vi "删除第一个元素.vi"(2 "数组－数值 2":dbl[](array[numeric]), 3 "数组－数值":dbl[](array[numeric])) -> (0 "数组－数值 3":dbl[](array[numeric]), 1 "数组":dbl[](array[numeric]))   [LabVIEW 2016]
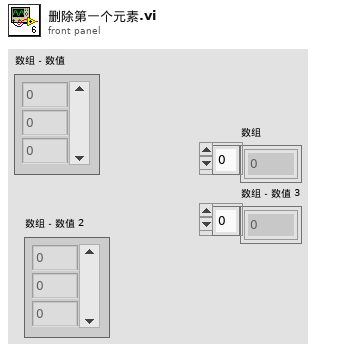
[diagram p1: front panel]
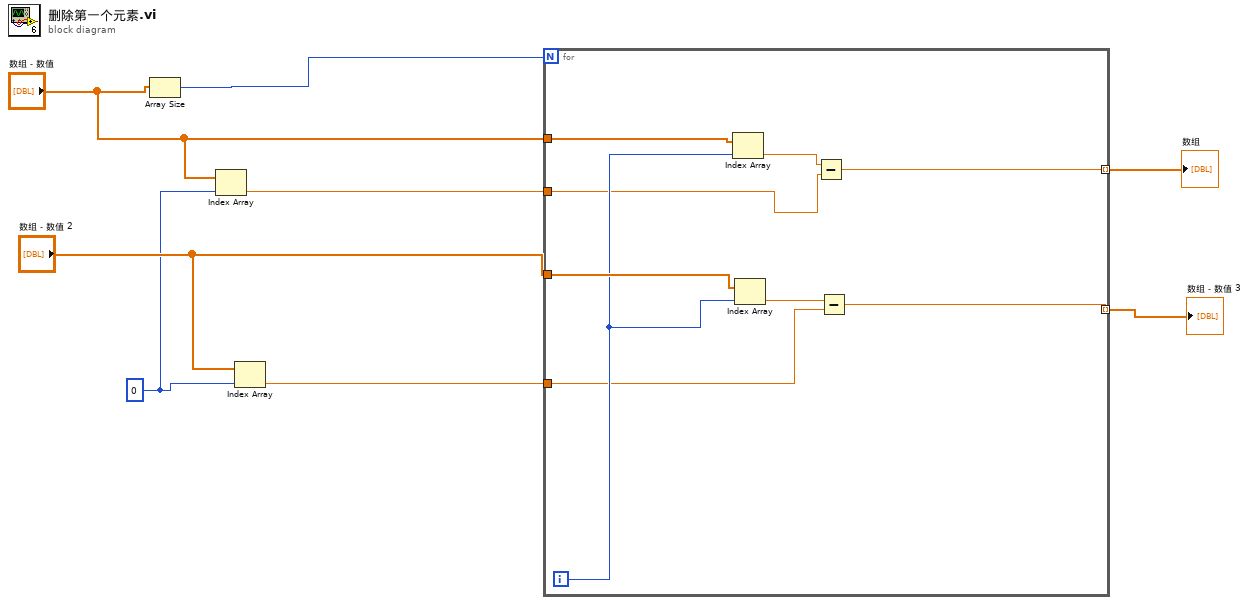
[diagram p0: block diagram]
diagram:
  w3 = 0 ("索引")
  n1 = Array Size(array="数组－数值") -> (size(s)=w5:i32)
  n2 = Index Array(array="数组－数值", index=w3) -> (element=w2:dbl)
  n3 = Index Array(array="数组－数值 2", index=w3) -> (element=w6:dbl)
  n4 = for {
    N: w5 -> [_]
    tunnel: "数组－数值" -> [w17]
    tunnel: "数组－数值 2" -> [w16]
    tunnel: [w12] -> w8 mode=indexing
    tunnel: [w11] -> w1 mode=indexing
    tunnel: w6 -> [w10]
    tunnel: w2 -> [w9]
    i -> [w15]
    n5 = Index Array(array=w17, index=w15) -> (element=w14:dbl)
    n6 = Index Array(array=w16, index=w15) -> (element=w13:dbl)
    n7 = Subtract(x=w14, y=w9) -> (x-y=w12:dbl)
    n8 = Subtract(x=w13, y=w10) -> (x-y=w11:dbl)
  }
  "数组" <- w8
  "数组－数值 3" <- w1
